vi "Simple Dependency Inspector.vi"(8 "error in":errorcluster) -> (0 "error out":errorcluster)   [LabVIEW 2020]
uses:
  Libraries/SimpleDependencyInspector/SimpleDependencyInspector.lvlib
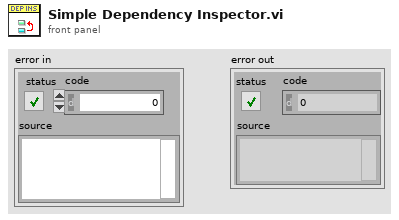
[diagram p1: front panel]
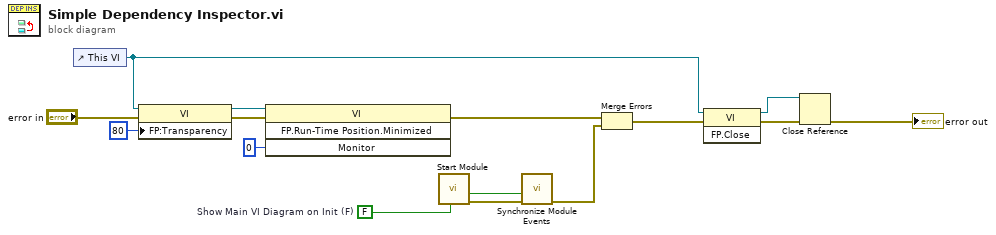
[diagram p0: block diagram]
diagram:
  w6 = FALSE  # Show Main VI Diagram on Init (F)
  n1 = control-ref of="This VI"() -> (w2:refnum<vi>)
  n2 = property class="VI"(reference=w2, error in="error in", "FP:Transparency"=u8 80 ("Front Panel Window:Transparency")) -> (reference out=w3:refnum<vi>, error out=w12:errorcluster)
  n3 = invoke class="VI" method="FP.Run-Time Position.Minimized"(reference=w3, error in=w12, "Monitor"=i16 0) -> (error out=w13:errorcluster)  [unwired: 1 in, 3 out]
  n4 = call "Start Module.vi"("Show Main VI Diagram on Init (F)"=w6) -> ("error out"=w15:errorcluster, "Wait for Event Sync?"=w7:bool)  [unwired: 7 in, 2 out]
  n5 = call "Synchronize Module Events.vi"("error in"=w15, "Wait for Event Sync?"=w7) -> ("error out"=w11:errorcluster)  [unwired: 9 in]
  n6 = Merge Errors(w13, w11) -> (w8:errorcluster)
  n7 = invoke class="VI" method="FP.Close"(reference=w2, error in=w8) -> (reference out=w1:refnum<vi>, error out=w14:errorcluster)  [unwired: 1 in, 1 out]
  n8 = Close Reference(reference=w1, error in (no error)=w14) -> (error out=→"error out":errorcluster)
